vi "String Word Wrap.vi"(9 "Max width (60)":i32=60, 11 "String in":string) -> (1 "Number of lines":i32, 3 "Wrapped lines":string[](array[string]))   [LabVIEW 2014, in "C Header Generator.lvlib"]
uses:
  C Header Generator.lvlib
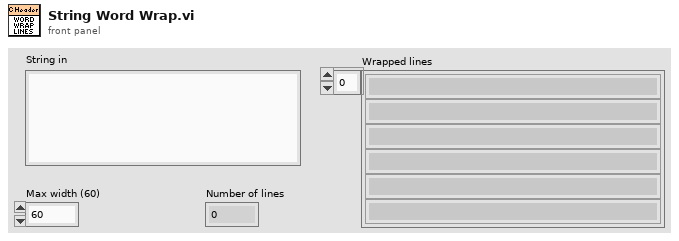
[diagram p1: front panel]
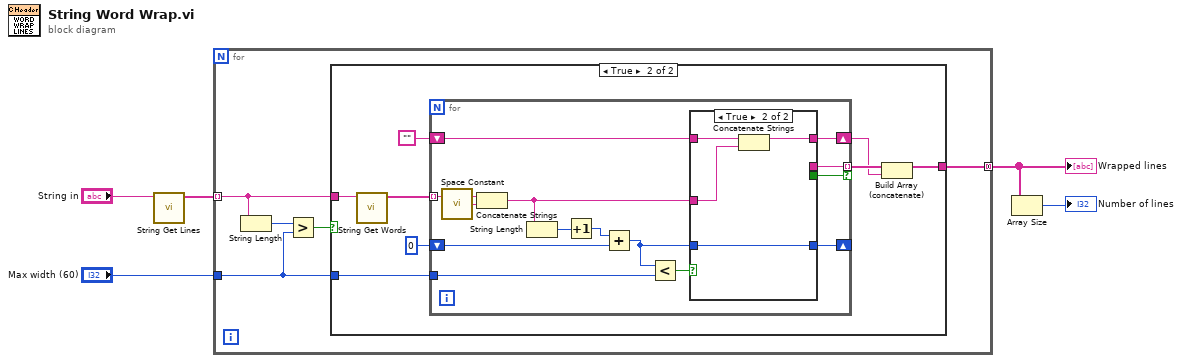
[diagram p0: block diagram]
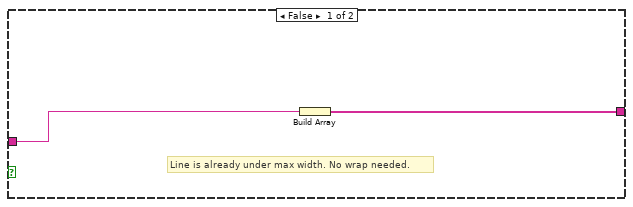
[diagram p2: hidden frame]
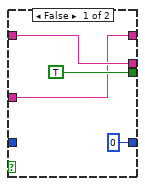
[diagram p3: hidden frame]
diagram:
  n1 = call "String Get Lines.vi"("string"="String in") -> ("lines"=w4:string[])  [unwired: 9 in, 1 out]
  n2 = for {
    tunnel: w4 -> [w8] mode=indexing
    tunnel: "Max width (60)" -> [w7]
    tunnel: [w6] -> w2 mode=concatenating
    n3 = String Length(string=w8) -> (length=w10:i32)
    n4 = Greater?(x=w10, y=w7) -> (0:w9:bool)
    n5 = case shown="True" w9 {
      tunnel: w8 -> [w12 w20]
      tunnel: w7 -> [_ w17]
      tunnel: [w11 w13] -> w6
      frame False {
        # "Line is already under max width. No wrap needed."
        n6 = Build Array(w12) -> (w11:string[])
      }
      frame True {
        n7 = call "String Get Words.vi"("input string"=w20) -> ("words"=w19:string[])  [unwired: 10 in]
        n8 = for {
          tunnel: w19 -> [w31] mode=indexing
          shift-right: [w26] -> _
          shift-left: 0 -> [w33]
          tunnel: w17 -> [w29]
          shift-right: [w23] -> w14
          shift-left: "" -> [w24]
          tunnel: [w22] -> w15 mode=indexing if=w21
          n9 = call <vilib>:"Space Constant.vi"() -> ("String"=w30:string)
          n10 = Concatenate Strings(w31, w30) -> (w25:string)
          n11 = String Length(string=w25) -> (length=w34:i32)
          n12 = Increment(x=w34) -> (x+1=w32:i32)
          n13 = Add(x=w32, y=w33) -> (x+y=w28:i32)
          n14 = Less?(x=w28, y=w29) -> (x < y?=w27:bool)
          n15 = case shown="True" w27 {
            tunnel: w24 -> [w38 w42]
            tunnel: w28 -> [_ w41]
            tunnel: [0 w41] -> w26
            tunnel: w25 -> [w36 w39]
            tunnel: [w36 w40] -> w23
            tunnel: [w38 _] -> w22
            tunnel: [TRUE _] -> w21
            frame False {
            }
            frame True {
              n16 = Concatenate Strings(w42, w39) -> (w40:string)
            }
          }
        }
        n17 = Build Array (concatenate)(w15, w14) -> (w13:string[])
      }
    }
  }
  "Wrapped lines" <- w2
  n18 = Array Size(array=w2) -> (size(s)=→"Number of lines":i32)
